vi "LSX Get Controller Call.vi"(8 "error in (no error)":errorcluster, 10 "plCtrCall":i32, 11 "lLSID":i32) -> (0 "error out":errorcluster, 2 "plCtrCall out":i32, 3 "function return":i32)   [LabVIEW 2018, in "Tango.lvlib"]
doc: "TANGOAPI int TANGOCALL LSX_GetControllerCall (int lLSID, int *plCtrCall);"
uses:
  Tango.lvlib
  SubVIs/Tango_DLL.dll
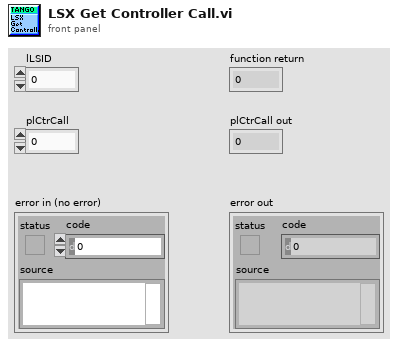
[diagram p1: front panel]
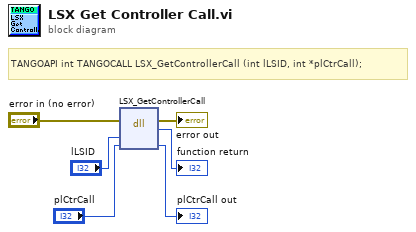
[diagram p0: block diagram]
diagram:
  # "TANGOAPI int TANGOCALL LSX_GetControllerCall (int lLSID, int *plCtrCall);"
  n1 = dll-call lib="C:/Users/Familie/Documents/LabviewIX81/lib/TANGO Stage/SubVIs/Tango_DLL.*" fn="LSX_GetControllerCall"(error in="error in (no error)", "lLSID"="lLSID", "plCtrCall"="plCtrCall") -> (error out=→"error out":errorcluster, →"function return":i32, "plCtrCall"=→"plCtrCall out":i32)  [unwired: 3 in, 1 out]
